vi "ShowScrollBar.vi"(8 "Origin in":T1, 9 "Task":enum16{"Read", "Open", "Close", "Reset"}(ring)=enum."Close", 11 "VI in":refnum<vi>) -> (0 "Origin":T1)   [LabVIEW 2019]
uses:
  <vilib>/Utility/miscctls.llb/LVPointTypeDef.ctl
  <vilib>/Utility/miscctls.llb/LVRectTypeDef.ctl
panel:
  out "InitialBounds":T2
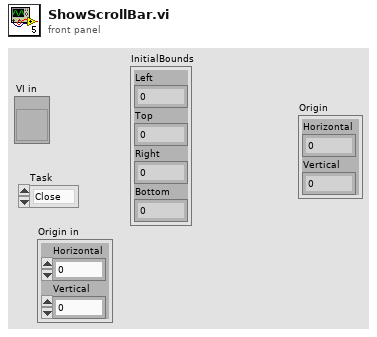
[diagram p1: front panel]
types:
  T1 = typedef "LVPointTypeDef.ctl" = cluster{"Horizontal":i16, "Vertical":i16}
  T2 = typedef "LVRectTypeDef.ctl" = cluster{"Left":i16, "Top":i16, "Right":i16, "Bottom":i16}
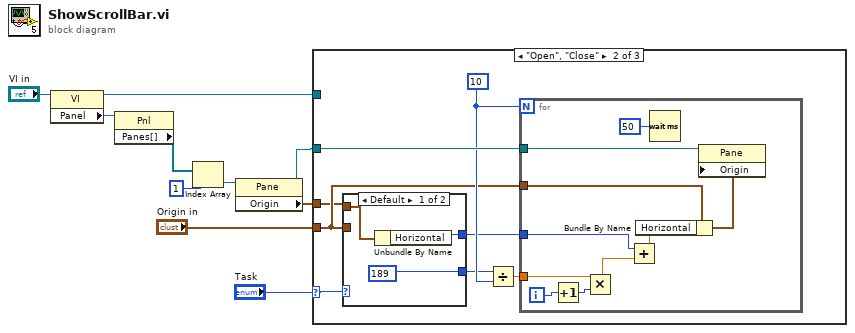
[diagram p0: block diagram]
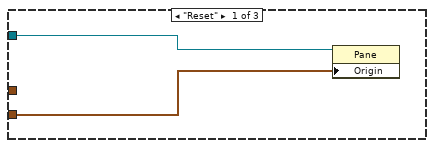
[diagram p2: hidden frame]
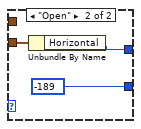
[diagram p3: hidden frame]
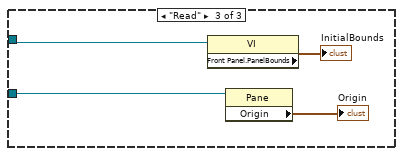
[diagram p4: hidden frame]
diagram:
  n1 = property class="VI"(reference="VI in") -> (reference out=w7:refnum<vi>, "Panel"=w8:refnum<vi>)  [unwired: 1 in, 1 out]
  n2 = property class="Pnl"(reference=w8) -> ("Panes[]"=w9:refnum<vi>[])  [unwired: 1 in, 2 out]
  n3 = Index Array(array=w9, index=1) -> (element=w2:refnum<vi>)
  n4 = property class="Pane"(reference=w2) -> (reference out=w1:refnum<vi>, "Origin"=w3:T1)  [unwired: 1 in, 1 out]
  n5 = case shown="\"Open\", \"Close\"" "Task" {
    selector: "Task" -> [_ w16 _]
    tunnel: w1 -> [w12 w20 w40]
    tunnel: w7 -> [_ _ w39]
    tunnel: "Origin in" -> [w11 w14 _]
    tunnel: w3 -> [_ w13 _]
    frame "Reset" {
      n6 = property class="Pane"(reference=w12, "Origin"=w11) -> ()  [unwired: 1 in, 2 out]
    }
    frame "Open", "Close" {
      w19 = 10
      n7 = case shown="Default" w16 {
        tunnel: [i16 189 ("y") i16 -189 ("y")] -> w17
        tunnel: [w21 w25] -> w15
        tunnel: w14 -> [_ w24]
        tunnel: w13 -> [w22 _]
        frame Default {
          n8 = Unbundle By Name(w22) -> ("Horizontal"=w21:i16)
        }
        frame "Open" {
          n9 = Unbundle By Name(w24) -> ("Horizontal"=w25:i16)
        }
      }
      n10 = Divide(x=w17, y=w19) -> (x/y=w18:dbl)
      n11 = for {
        N: w19 -> [_]
        tunnel: w20 -> [w36]
        tunnel: w18 -> [w30]
        tunnel: w14 -> [w32]
        tunnel: w15 -> [w27]
        i -> [w31]
        n12 = Increment(x=w31) -> (x+1=w28:i32)
        n13 = Multiply(x=w30, y=w28) -> (x*y=w29:dbl)
        n14 = Add(x=w27, y=w29) -> (x+y=w33:dbl)
        n15 = Bundle By Name(cluster=w32, "Horizontal"=w33) -> (w35:T1)
        n16 = Wait (ms)(milliseconds to wait=u32 50) -> ()  [unwired: 1 out]
        n17 = property class="Pane"(reference=w36, "Origin"=w35) -> ()  [unwired: 1 in, 2 out]
      }
    }
    frame "Read" {
      n18 = property class="VI"(reference=w39) -> ("Front Panel.PanelBounds"=→"InitialBounds":T2)  [unwired: 1 in, 2 out]
      n19 = property class="Pane"(reference=w40) -> ("Origin"=→"Origin":T1)  [unwired: 1 in, 2 out]
    }
  }
